vi "Write event data.vi"(8 "error in (no error)":errorcluster, 10 "Update DT":T1, 11 "Update DT Event Msg in":refnum<class "Update DT Event Msg.lvclass">) -> (0 "error out":errorcluster, 3 "Update DT Event Msg out":refnum<class "Update DT Event Msg.lvclass">)   [LabVIEW 2016, in "Controller UI.lvlib" / "Update DT Event Msg.lvclass"]
uses:
  <userlib>/Common Components/Controller UI Messages/Update DT Event Msg/Update DT Event Msg.lvclass
  <userlib>/Common Components/Controller UI/Update DT event data.ctl
  <userlib>/Common Components/Controller UI/Update DT Cmd.ctl
  <userlib>/Common Components/Controller UI Messages/Update DT Event Msg/Update DT Event Msg.lvclass/Update DT Event Msg.ctl
  <userlib>/Common Components/Controller UI/Controller UI.lvclass
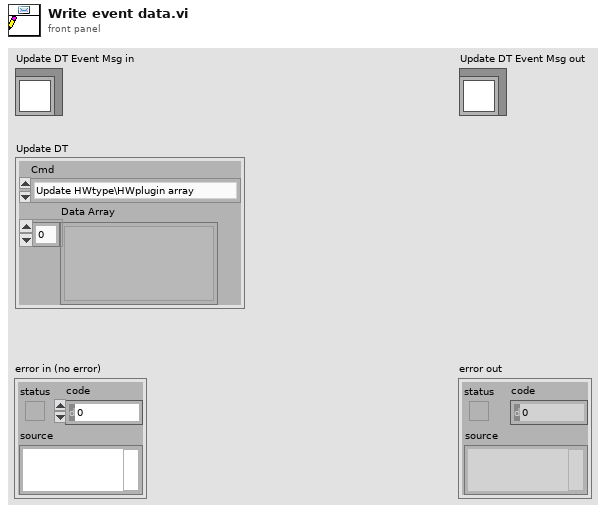
[diagram p1: front panel]
types:
  T1 = typedef "Controller UI.lvlib/Controller UI.lvclass/Update DT event data.ctl" = cluster{"Cmd":T2, "Data Array":variant[]}
  T2 = typedef "Controller UI.lvlib/Controller UI.lvclass/Update DT Cmd.ctl" = enum16{"Update HWtype\\HWplugin array", "Update Checked-out", "Update COMM Status", "Load DevInfo from File", "Save DevInfo to File", "Update COMM Address List"}
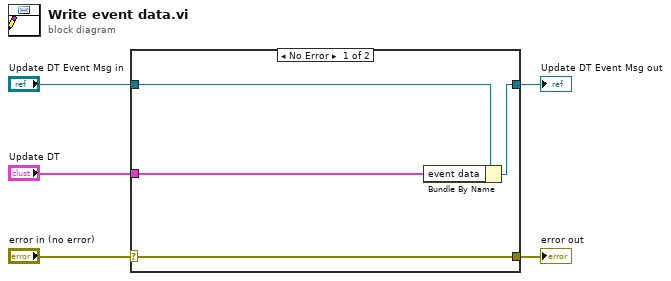
[diagram p0: block diagram]
diagram:
  n1 = case shown="No Error" "error in (no error)" {
    selector: "error in (no error)" -> [w9 w10]
    tunnel: [w9 w10] -> w4
    tunnel: [w7 w11] -> w2
    tunnel: "Update DT Event Msg in" -> [w8 w11]
    tunnel: "Update DT" -> [w6 _]
    frame No Error {
      n2 = Bundle By Name(cluster=w8, "event data"=w6) -> (w7:refnum<class "Update DT Event Msg.lvclass">)
    }
    frame Error {
    }
  }
  "error out" <- w4
  "Update DT Event Msg out" <- w2
